vi "driveCommandCreator.vi"(4 "JoystickDevRef 2":T1, 6 "JoystickDevRef":T1, 8 "toFreestyle":bool, 9 "toDriveDistance":bool, 10 "toTurnAngle":bool, 11 "toDoNothing":bool) -> ()   [LabVIEW 2017]
uses:
  <vilib>/Rock Robotics/WPI/Joystick/WPI_JoystickDevRef.ctl
  <vilib>/Rock Robotics/WPI/Joystick/WPI_JoystickDeviceEnum.ctl
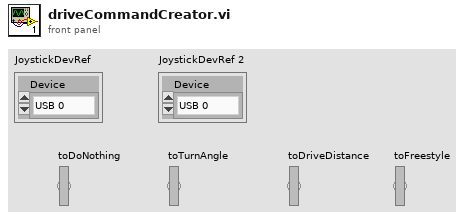
[diagram p1: front panel]
types:
  T1 = typedef "WPI_JoystickDevRef.ctl" = cluster{"Device":T2}
  T2 = typedef "WPI_JoystickDeviceEnum.ctl" = enum16{"USB 0", "USB 1", "USB 2", "USB 3", "USB 4", "USB 5"}
  T3 = typedef "driveLogicStates.ctl" = enum16{"doNothing", "driveDistance", "turnAngle", "freestyle", "guidedDrive", "approachingElement"}
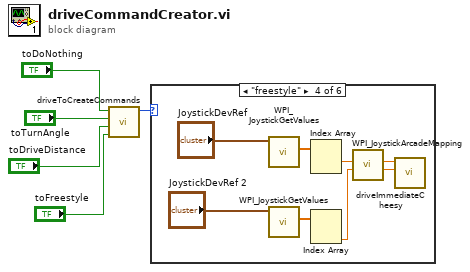
[diagram p0: block diagram]
diagram:
  n1 = call "driveToCreateCommands.vi"("toFreestyle"="toFreestyle", "toDriveDistance"="toDriveDistance", "toTurnAngle"="toTurnAngle", "toDoNothing"="toDoNothing") -> ("Current state"=w1:T3)  [unwired: 7 in]
  n2 = case shown="\"freestyle\"" w1 {
    frame "doNothing", Default {
    }
    frame "driveDistance" {
    }
    frame "turnAngle" {
    }
    frame "freestyle" {
      n3 = call <vilib>:"WPI_JoystickGetValues.vi"("JoystickDevRef"="JoystickDevRef") -> ("Axes"=w13:dbl[])  [unwired: 6 in, 4 out]
      n4 = call <vilib>:"WPI_JoystickGetValues.vi"("JoystickDevRef"="JoystickDevRef 2") -> ("Axes"=w12:dbl[])  [unwired: 6 in, 4 out]
      n5 = Index Array(array=w13) -> (element #1=w11:dbl)  [unwired: 2 in, 1 out]
      n6 = Index Array(array=w12) -> (element #2=w10:dbl)  [unwired: 2 in, 1 out]
      n7 = call <vilib>:"WPI_JoystickArcadeMapping.vi"("Y axis value"=w10, "X axis value"=w11) -> ("Right Motor Value"=w8:dbl, "Left Motor Value"=w9:dbl)  [unwired: 8 in]
      n8 = call "driveImmediateCheesy.vi"("Right Motor"=w8, "Left Motor"=w9) -> ()  [unwired: 9 in, 1 out]
    }
    frame "guidedDrive" {
    }
    frame "approachingElement" {
    }
  }
